vi "Connect ROV.vi"(6 "Teleop command":T1={"Motor command"=[0, 0, 0, 0, 0, 0]}, 7 "IP address":string="XXX.XXX.XXX.XXX", 8 "error in (no error)":errorcluster, 11 "connection ID":refnum<k16>) -> (0 "error out":errorcluster, 3 "connection ID out":refnum<k16>)   [LabVIEW 2012]
doc: "This VI uses the connection ID to send the Teleop command via UDP so that only the most recent message is read and processed on the ROV. The Teleop command is flattened to a string incoded in HEX as the 'UDP Write' function expects and is transmitted to the specified IP address.\nRuffin"
uses:
  Teleop command.ctl
  Support/Robot globals (robot acquires video).vi
  Support/Host globals (robot acquires video).vi
  ROV Host.lvclass
panel:
  out "data string":string
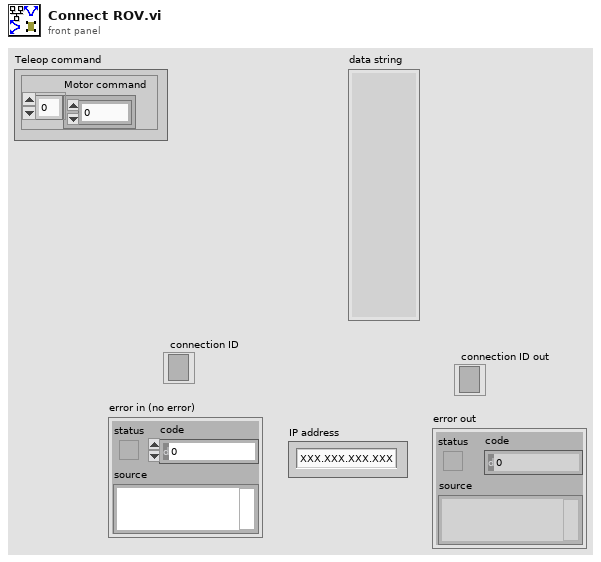
[diagram p1: front panel]
types:
  T1 = typedef "ROV Host.lvclass/Teleop command.ctl" = cluster{"Motor command":i8[]}
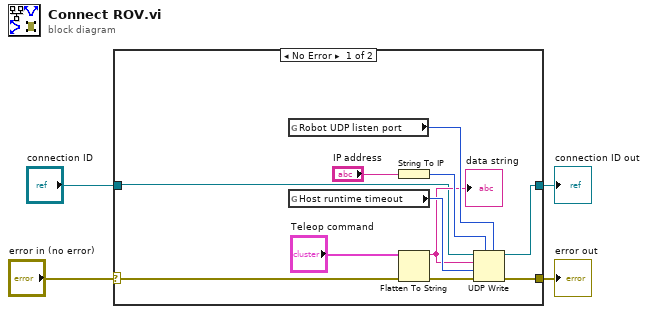
[diagram p0: block diagram]
diagram:
  n1 = case shown="No Error" "error in (no error)" {
    selector: "error in (no error)" -> [w8 w16]
    tunnel: "connection ID" -> [w7 w17]
    tunnel: [w6 w17] -> w2
    tunnel: [w5 w16] -> w1
    frame No Error {
      n2 = global read "Robot globals (robot acquires video).vi" "Robot UDP listen port"() -> (w14:u16)
      n3 = global read "Host globals (robot acquires video).vi" "Host runtime timeout"() -> (w15:i32)
      n4 = String To IP(1:"IP address") -> (0:w12:u32)
      n5 = Flatten To String(anything="Teleop command", error in (no error)=w8) -> (data string=w9:string, error out=w10:errorcluster)  [unwired: 2 in, 1 out]
      "data string" <- w9
      n6 = UDP Write(address=w12, port or service name=w14, connection ID=w7, data in=w9, 8:w10, 9:w15) -> (error out=w5:errorcluster, 3:w6:refnum<k16>)
    }
    frame Error {
    }
  }
  "error out" <- w1
  "connection ID out" <- w2
